vi "MoveWithVelocity.vi"(0 "axis in":cluster{"keyHandle":u32, "nodeId":u16}={"keyHandle"=0, "nodeId"=1}, 5 "velocity profile":T1, 7 "targetVelocity":i32, 9 "timeout":u32, 11 "error in (no error)":errorcluster) -> (4 "axis out":cluster{"keyHandle":u32, "nodeId":u16}={"keyHandle"=0, "nodeId"=1}, 15 "error out":errorcluster)   [LabVIEW 2019]
doc: "<B>MoveWithVelocity</B> starts the movement with a defined velocity. Before the movement starts, the velocity profile is written."
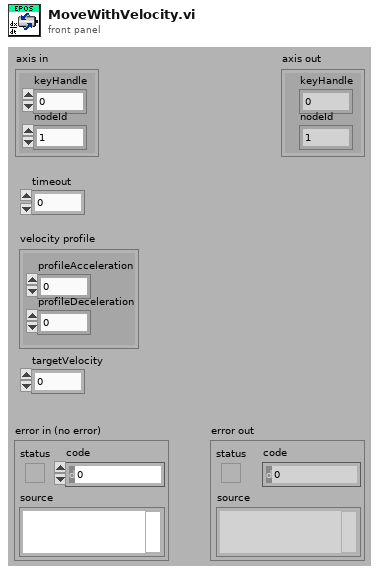
[diagram p1: front panel]
types:
  T1 = cluster{"profileAcceleration":u32, "profileDeceleration":u32}
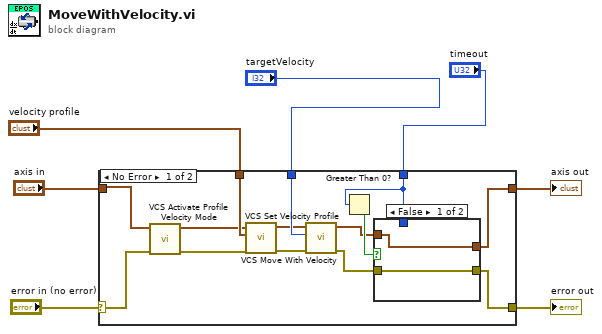
[diagram p0: block diagram]
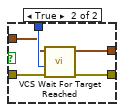
[diagram p2: hidden frame]
diagram:
  n1 = case shown="No Error" "error in (no error)" {
    selector: "error in (no error)" -> [w8 w30]
    tunnel: [w12 w30] -> w6
    tunnel: [w13 w29] -> w5
    tunnel: "axis in" -> [w9 w29]
    tunnel: "targetVelocity" -> [w21 _]
    tunnel: "velocity profile" -> [w20 _]
    tunnel: "timeout" -> [w17 _]
    frame No Error {
      n2 = call "VCS Activate Profile Velocity Mode.vi"("error in (no error)"=w8, "axis in"=w9) -> ("error out"=w11:errorcluster, "axis out"=w10:cluster{"keyHandle":u32, "nodeId":u16})  [unwired: 8 in]
      n3 = call "VCS Set Velocity Profile.vi"("error in (no error)"=w11, "velocity profile"=w20, "axis in"=w10) -> ("error out"=w18:errorcluster, "axis out"=w19:cluster{"keyHandle":u32, "nodeId":u16})  [unwired: 7 in]
      n4 = call "VCS Move With Velocity.vi"("error in (no error)"=w18, "targetVelocity"=w21, "axis in"=w19) -> ("error out"=w14:errorcluster, "axis out"=w15:cluster{"keyHandle":u32, "nodeId":u16})  [unwired: 7 in]
      n5 = Greater Than 0?(x=w17) -> (x > 0?=w16:bool)
      n6 = case shown="False" w16 {
        tunnel: [w23 w28] -> w13
        tunnel: [w22 w27] -> w12
        tunnel: w17 -> [_ w26]
        tunnel: w15 -> [w23 w25]
        tunnel: w14 -> [w22 w24]
        frame False {
        }
        frame True {
          n7 = call "VCS Wait For Target Reached.vi"("error in (no error)"=w24, "timeout"=w26, "axis in"=w25) -> ("error out"=w27:errorcluster, "axis out"=w28:cluster{"keyHandle":u32, "nodeId":u16})  [unwired: 7 in]
        }
      }
    }
    frame Error {
    }
  }
  "error out" <- w6
  "axis out" <- w5
